vi "Solve_Correspondance_Problem-5.vi"(0 "[IN] Indicies of Po\nints Inside Trks":i32[](array[numeric]), 1 "[IN] Subtracks":T3(array[cluster]), 3 "[IN] Still connected\ntracks in group":T2, 5 "[IN] Indicies of all \nAffected Tracks \n(initial point = 0)":i32[](array[numeric]), 7 "[IN] Index of Optimal \nSubtrack Splitting Case":i32, 9 "[IN] Optimal solution \nfor Merging Case":i32[](array[numeric]), 11 "error IN":errorcluster, 12 "[IN] Status of 1st \nProblem Point":i16) -> (4 "[OUT] Clusters for Re\nconstructed Tracks":T1, 15 "error OUT":errorcluster)   [LabVIEW 2013]
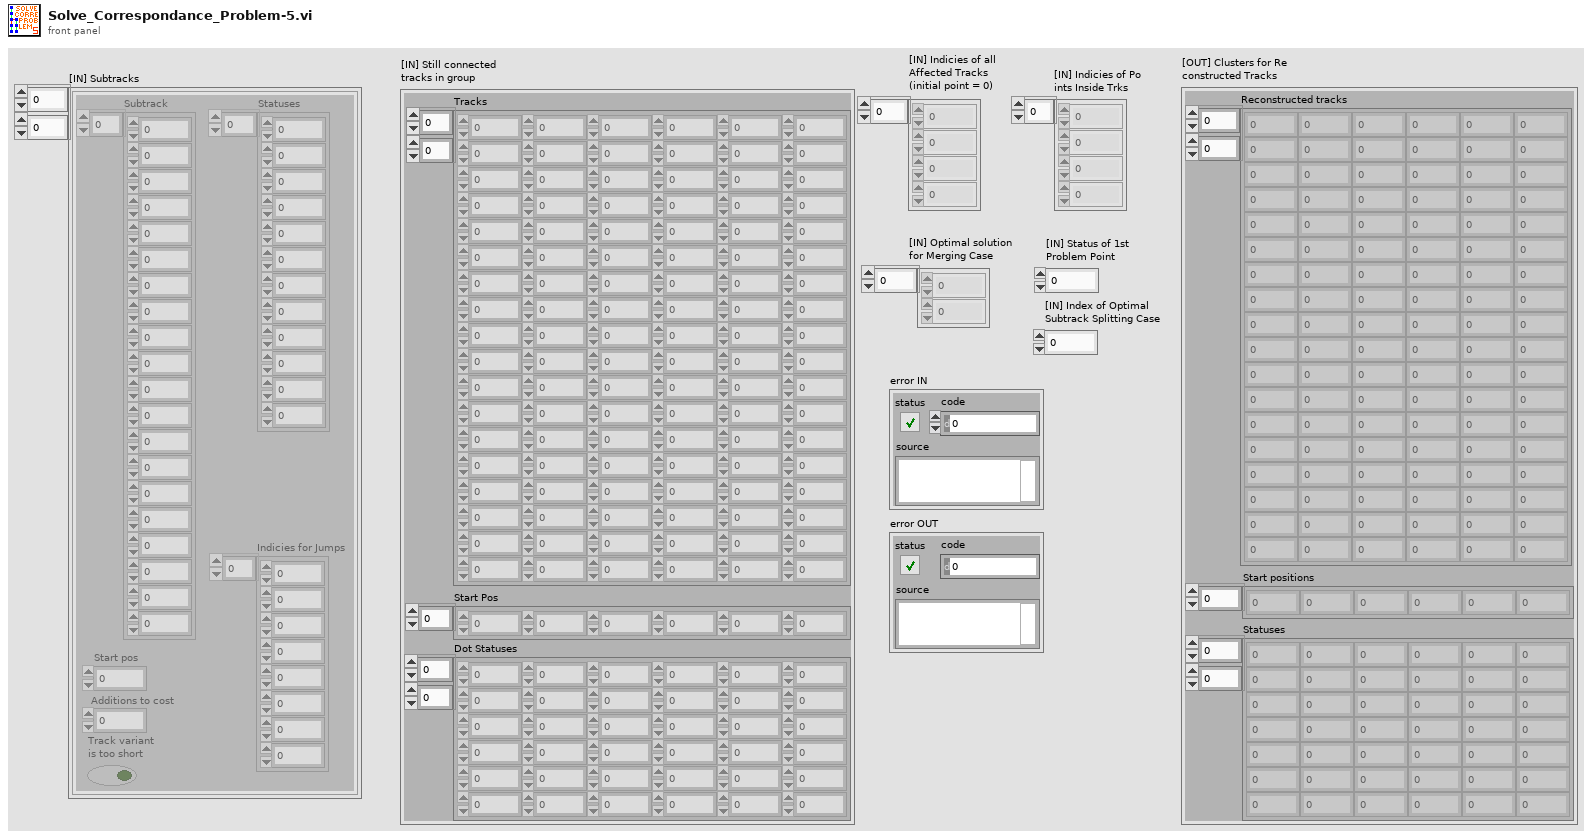
[diagram p1: front panel]
types:
  T1 = cluster{"Reconstructed tracks":dbl[][], "Start positions":i32[], "Statuses":i16[][]}
  T2 = cluster{"Tracks":dbl[][], "Start Pos":i32[], "Dot Statuses":i16[][]}
  T3 = cluster{"Subtrack":dbl[], "Statuses":i16[], "Start pos":i32, "Additions to cost":i8, "Track variant \nis too short":bool, "Indicies for Jumps":i32[]}[][]
  T4 = cluster{"Subtrack":dbl[], "Statuses":i16[], "Start pos":i32, "Additions to cost":i8, "Track variant \nis too short":bool, "Indicies for Jumps":i32[]}[]
  T5 = cluster{"Subtrack":dbl[], "Statuses":i16[], "Start pos":i32, "Additions to cost":i8, "Track variant \nis too short":bool, "Indicies for Jumps":i32[]}
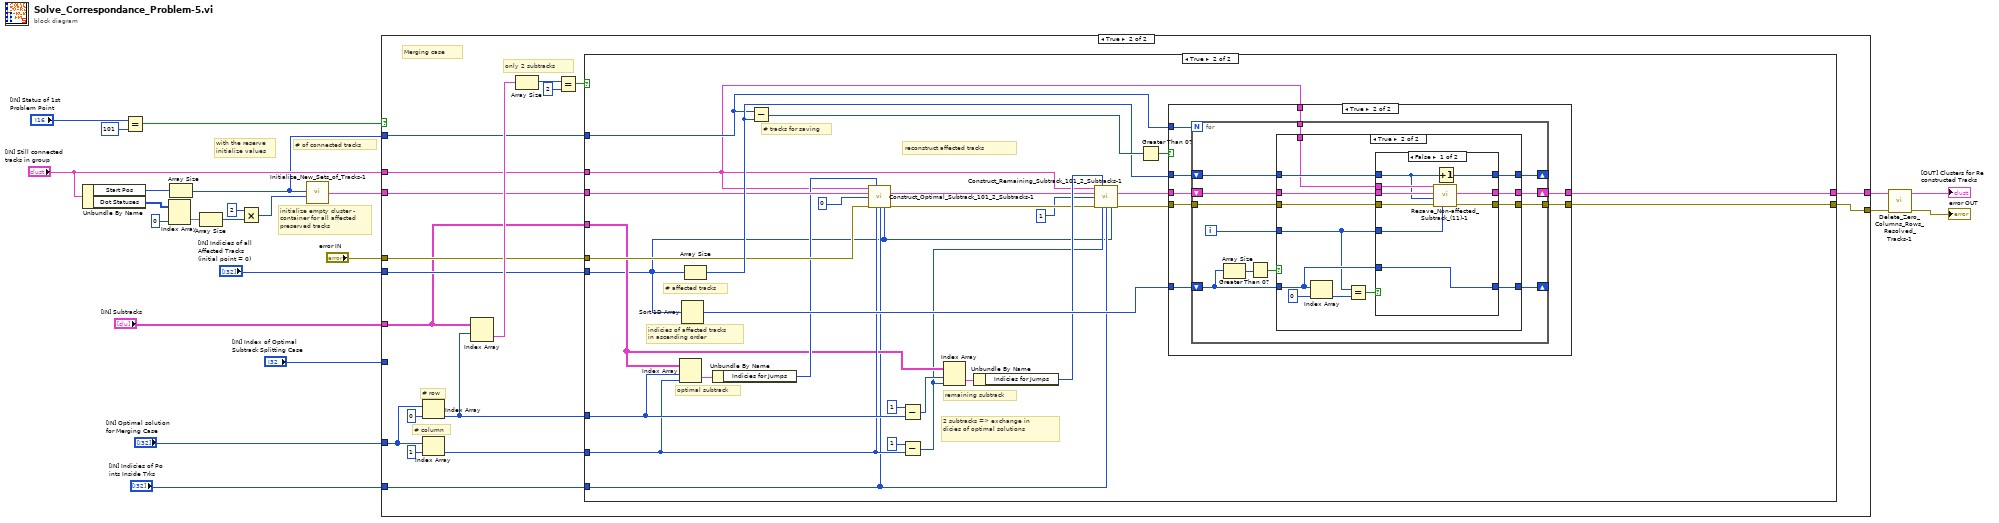
[diagram p0: block diagram]
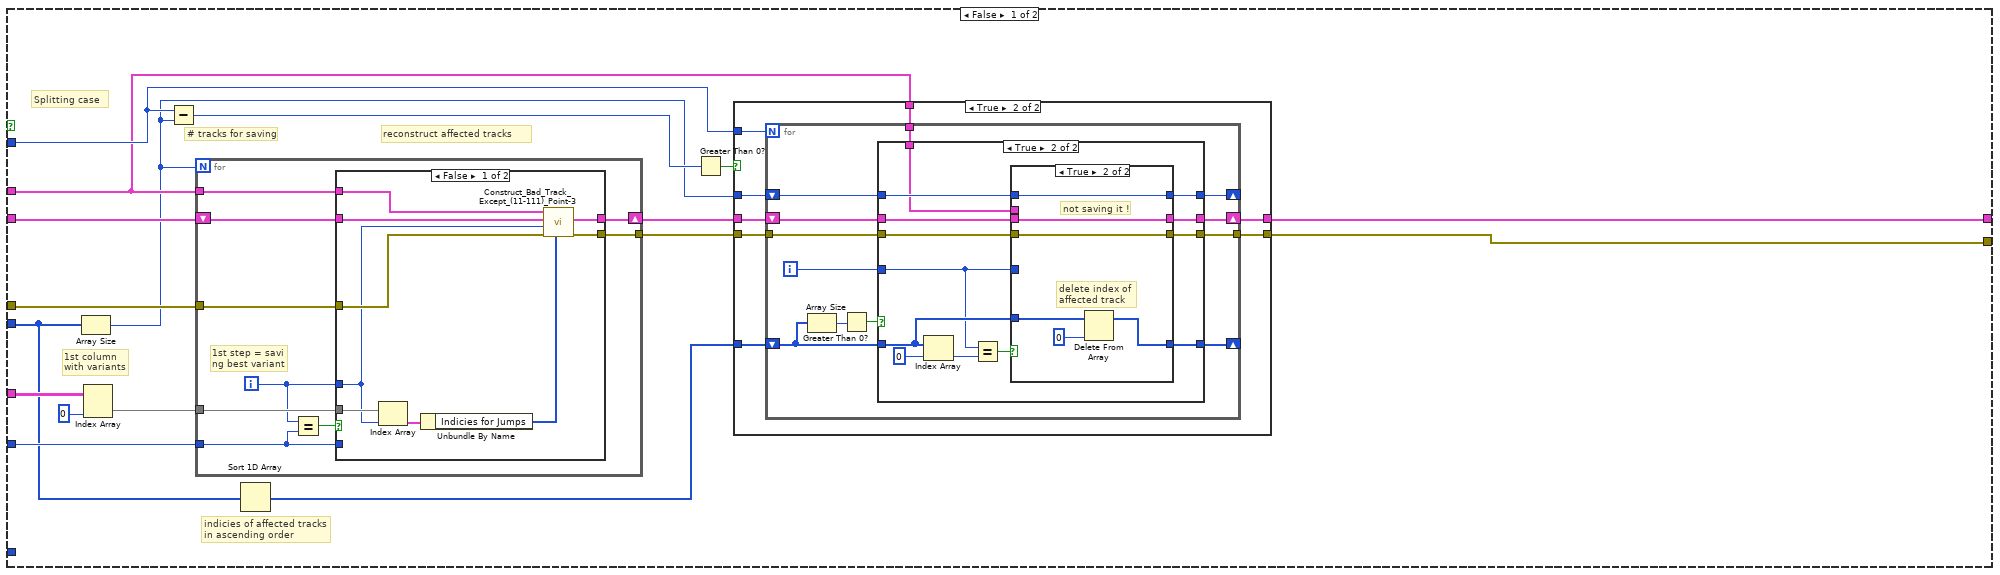
[diagram p2: hidden frame]
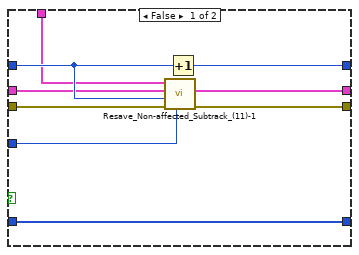
[diagram p4: hidden frame]
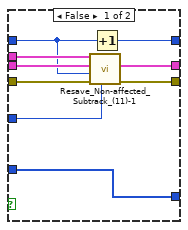
[diagram p5: hidden frame]
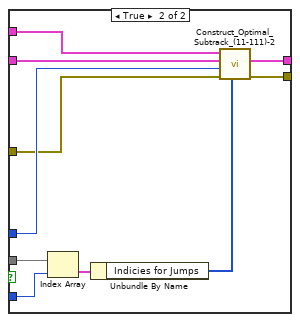
[diagram p6: hidden frame]
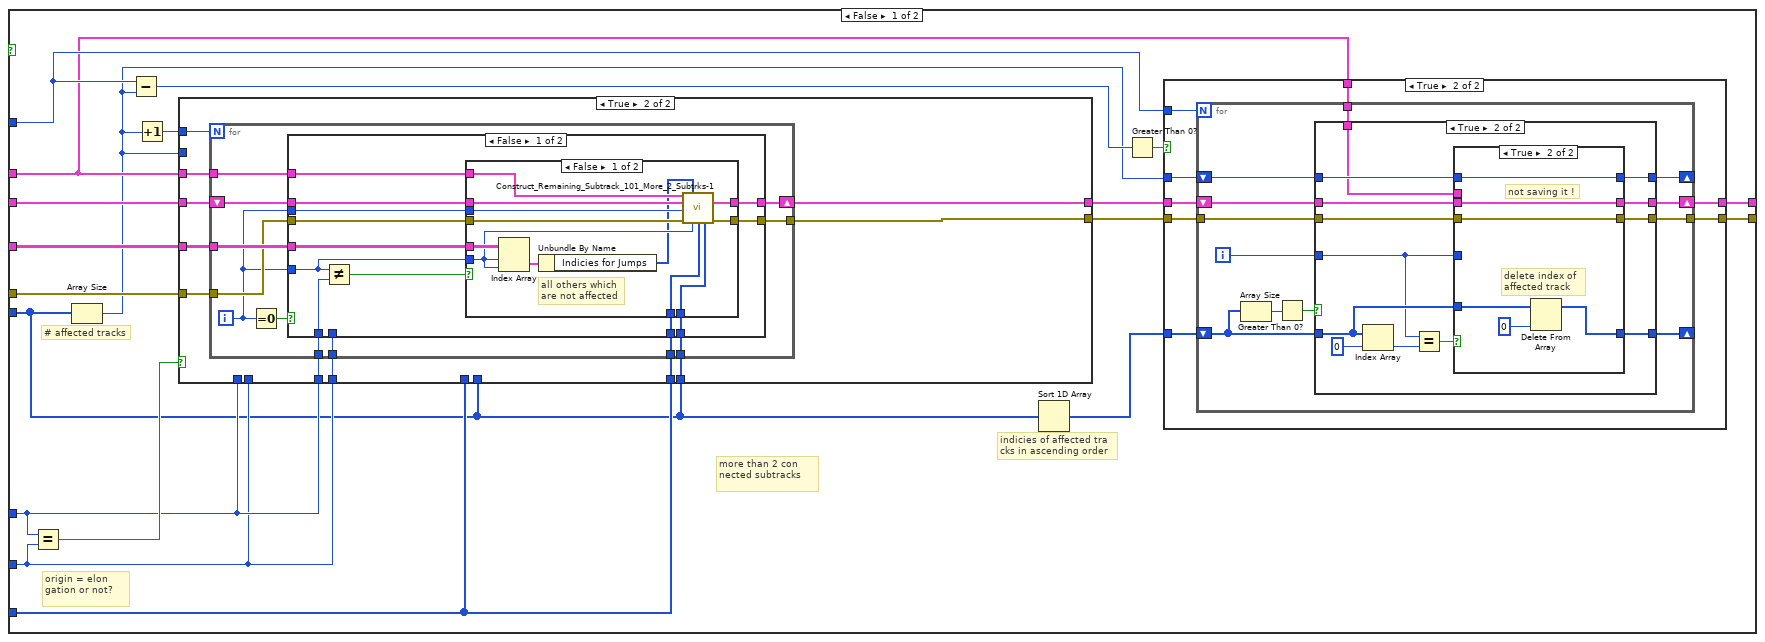
[diagram p7: hidden frame]
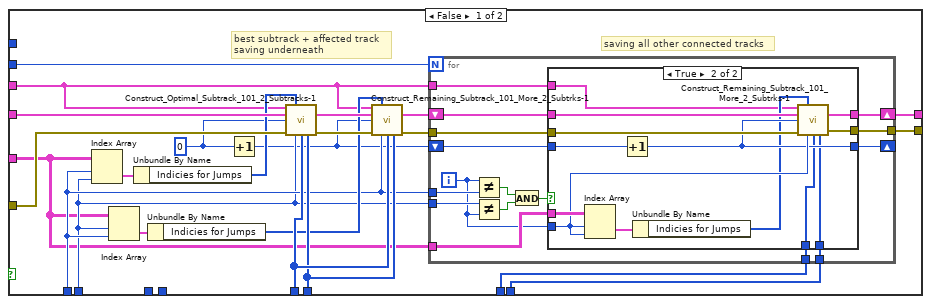
[diagram p8: hidden frame]
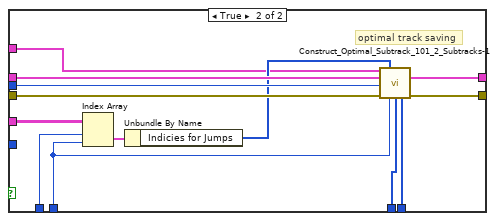
[diagram p11: hidden frame]
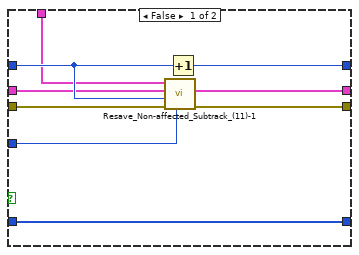
[diagram p13: hidden frame]
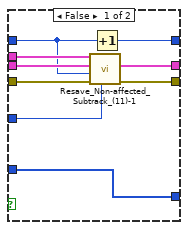
[diagram p14: hidden frame]
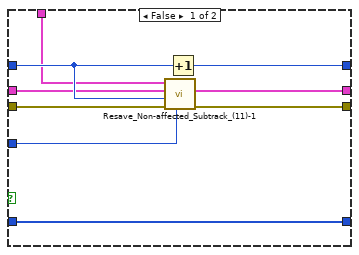
[diagram p16: hidden frame]
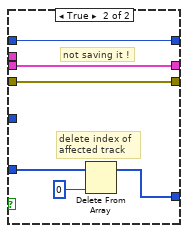
[diagram p17: hidden frame]
diagram:
  # "# of connected tracks"
  # "with the reserve\ninitialize values"
  # "initialize empty cluster - \ncontainer for all affected\npreserved tracks"
  n1 = Unbundle By Name("[IN] Still connected\ntracks in group") -> ("Start Pos"=w19:i32[], "Dot Statuses"=w8:i16[][])
  n2 = Equal?(x="[IN] Status of 1st \nProblem Point", y=i16 101) -> (x = y?=w21:bool)
  n3 = Index Array(array=w8, index (col)=0 ("disabled index (col)")) -> (element=w17:i16[])  [unwired: 1 in]
  n4 = Array Size(array=w19) -> (size(s)=w9:i32)
  n5 = Array Size(array=w17) -> (size(s)=w16:i32)
  n6 = Multiply(x=2, y=w16) -> (x*y=w7:i32)
  n7 = call "Initialize_New_Sets_of_Tracks-1.vi"("[IN] # of Eleme\nnts in New Tracks"=w7, "[IN] # previously \nconnected tracks"=w9) -> ("[OUT] Clusters for Re\nconstructed Tracks"=w14:T1)  [unwired: 4 in]
  n8 = case shown="True" w21 {
    tunnel: "[IN] Still connected\ntracks in group" -> [w27 w135]
    tunnel: w14 -> [w38 w138]
    tunnel: "[IN] Subtracks" -> [w40 w130]
    tunnel: "[IN] Indicies of all \nAffected Tracks \n(initial point = 0)" -> [w29 w136]
    tunnel: "[IN] Index of Optimal \nSubtrack Splitting Case" -> [w36 _]
    tunnel: "error IN" -> [w35 w134]
    tunnel: w9 -> [w30 w137]
    tunnel: [w25 w129] -> w6
    tunnel: [w24 w128] -> w5
    tunnel: "[IN] Optimal solution \nfor Merging Case" -> [_ w143]
    tunnel: "[IN] Indicies of Po\nints Inside Trks" -> [_ w133]
    frame False {
      # "indicies of affected tracks\nin ascending order"
      # "# tracks for saving"
      # "reconstruct affected tracks"
      # "1st column \nwith variants"
      # "Splitting case"
      n9 = Array Size(array=w29) -> (size(s)=w26:i32)
      n10 = Index Array(array=w40, index (col)=0 ("disabled index (col)")) -> (element=w37:T4)  [unwired: 1 in]
      n11 = Subtract(x=w30, y=w26) -> (x-y=w31:i32)
      n12 = for {
        N: w26 -> [_]
        shift-right: [w103] -> w34
        shift-left: w38 -> [w108]
        tunnel: w27 -> [w107]
        tunnel: w37 -> [w105]
        tunnel: w36 -> [w101]
        tunnel: w35 -> [w106]
        tunnel: [w104] -> w33
        i -> [w102]
        # "1st step = savi\nng best variant"
        n13 = Equal?(x=w102, y=w101) -> (x = y?=w100:bool)
        n14 = case shown="False" w100 {
          tunnel: w108 -> [w117 w123]
          tunnel: w107 -> [w116 w124]
          tunnel: w106 -> [w113 w121]
          tunnel: w102 -> [w109 w122]
          tunnel: w105 -> [w115 w127]
          tunnel: w101 -> [_ w126]
          tunnel: [w111 w118] -> w103
          tunnel: [w110 w119] -> w104
          frame False {
            n15 = Index Array(array=w115, index=w109) -> (element=w114:T5)
            n16 = Unbundle By Name(w114) -> ("Indicies for Jumps"=w112:i32[])
            n17 = call "Construct_Bad_Track_Except_(11-111)_Point-3.vi"("[IN] Indexes for Jumps"=w112, "error IN"=w113, "[IN] Index of recon\nstructed tracks"=w109, "[IN] Clusters for Re\nconstructed Tracks"=w117, "[IN] Still connected\ntracks in group"=w116) -> ("error OUT"=w110:errorcluster, "[OUT] Clusters for Re\nconstructed Tracks"=w111:T1)  [unwired: 5 in]
          }
          frame True {
            n18 = Index Array(array=w127, index=w126) -> (element=w125:T5)
            n19 = Unbundle By Name(w125) -> ("Indicies for Jumps"=w120:i32[])
            n20 = call "Construct_Optimal_Subtrack_(11-111)-2.vi"("[IN] Indexes for Jumps"=w120, "error IN"=w121, "[IN] Index of recon\nstructed tracks"=w122, "[IN] Clusters for Re\nconstructed Tracks"=w123, "[IN] Still connected\ntracks in group"=w124) -> ("error OUT"=w119:errorcluster, "[OUT] Clusters for Re\nconstructed Tracks"=w118:T1)  [unwired: 5 in]
          }
        }
      }
      n21 = Sort 1D Array(array=w29) -> (sorted array=w28:i32[])
      n22 = Greater Than 0?(x=w31) -> (x > 0?=w32:bool)
      n23 = case shown="True" w32 {
        tunnel: w34 -> [w42 w48]
        tunnel: w33 -> [w41 w47]
        tunnel: w30 -> [_ w50]
        tunnel: w28 -> [_ w49]
        tunnel: w27 -> [_ w45]
        tunnel: w26 -> [_ w46]
        tunnel: [w41 w44] -> w24
        tunnel: [w42 w43] -> w25
        frame False {
        }
        frame True {
          n24 = for {
            N: w50 -> [_]
            shift-right: [w51] -> _
            shift-left: w49 -> [w52]
            shift-right: [w54] -> w43
            shift-left: w48 -> [w58]
            tunnel: w47 -> [w57]
            shift-right: [w56] -> _
            shift-left: w46 -> [w59]
            tunnel: w45 -> [w55]
            tunnel: [w53] -> w44
            i -> [w60]
            n25 = Array Size(array=w52) -> (size(s)=w62:i32)
            n26 = Greater Than 0?(x=w62) -> (x > 0?=w61:bool)
            n27 = case shown="True" w61 {
              tunnel: w60 -> [w71 w72]
              tunnel: w59 -> [w70 w79]
              tunnel: w58 -> [w69 w81]
              tunnel: w57 -> [w67 w80]
              tunnel: [w68 w76] -> w56
              tunnel: w55 -> [w66 w73]
              tunnel: [w65 w78] -> w54
              tunnel: [w64 w77] -> w53
              tunnel: w52 -> [w63 w75]
              tunnel: [w63 w74] -> w51
              frame False {
                n28 = call "Resave_Non-affected_Subtrack_(11)-1.vi"("[IN] Index for Not\nAffected Track"=w71, "error IN"=w67, "[IN] Index of recon\nstructed tracks"=w70, "[IN] Clusters for Re\nconstructed Tracks"=w69, "[IN] Still connected\ntracks in group"=w66) -> ("error OUT"=w64:errorcluster, "[OUT] Clusters for Re\nconstructed Tracks"=w65:T1)  [unwired: 5 in]
                n29 = Increment(x=w70) -> (x+1=w68:i32)
              }
              frame True {
                n30 = Index Array(array=w75, index=0) -> (element=w83:i32)
                n31 = Equal?(x=w72, y=w83) -> (x = y?=w82:bool)
                n32 = case shown="True" w82 {
                  tunnel: w81 -> [w92 w99]
                  tunnel: w80 -> [w90 w98]
                  tunnel: w79 -> [w86 w97]
                  tunnel: [w88 w99] -> w78
                  tunnel: [w87 w98] -> w77
                  tunnel: [w89 w97] -> w76
                  tunnel: w75 -> [w93 w96]
                  tunnel: [w93 w94] -> w74
                  tunnel: w73 -> [w91 _]
                  tunnel: w72 -> [w85 _]
                  frame False {
                    n33 = call "Resave_Non-affected_Subtrack_(11)-1.vi"("[IN] Index for Not\nAffected Track"=w85, "error IN"=w90, "[IN] Index of recon\nstructed tracks"=w86, "[IN] Clusters for Re\nconstructed Tracks"=w92, "[IN] Still connected\ntracks in group"=w91) -> ("error OUT"=w87:errorcluster, "[OUT] Clusters for Re\nconstructed Tracks"=w88:T1)  [unwired: 5 in]
                    n34 = Increment(x=w86) -> (x+1=w89:i32)
                  }
                  frame True {
                    # "not saving it !"
                    # "delete index of \naffected track"
                    n35 = Delete From Array(array=w96, index=0) -> (array with subset deleted=w94:i32[])  [unwired: 1 in, 1 out]
                  }
                }
              }
            }
          }
        }
      }
    }
    frame True {
      # "Merging case"
      # "only 2 subtracks"
      # "# column"
      # "# row"
      n36 = Index Array(array=w143, index=0) -> (element=w131:i32)
      n37 = Index Array(array=w143, index=1) -> (element=w132:i32)
      n38 = Index Array(array=w130, index (row)=w131) -> (element=w142:T4)  [unwired: 1 in]
      n39 = Array Size(array=w142) -> (size(s)=w141:i32)
      n40 = Equal?(x=w141, y=2) -> (x = y?=w139:bool)
      n41 = case shown="True" w139 {
        tunnel: w138 -> [w156 w364]
        tunnel: w135 -> [w157 w348]
        tunnel: w137 -> [w161 w365]
        tunnel: w136 -> [w147 w343]
        tunnel: w134 -> [w158 w362]
        tunnel: w133 -> [w149 w344]
        tunnel: w132 -> [w150 w354]
        tunnel: w131 -> [w151 w356]
        tunnel: w130 -> [w155 w353]
        tunnel: [w163 w361] -> w129
        tunnel: [w162 w360] -> w128
        frame False {
          # "indicies of affected tra\ncks in ascending order"
          # "origin = elon\ngation or not?"
          # "# affected tracks"
          # "more than 2 con\nnected subtracks"
          n42 = Equal?(x=w151, y=w150) -> (x = y?=w159:bool)
          n43 = Array Size(array=w147) -> (size(s)=w148:i32)
          n44 = Subtract(x=w161, y=w148) -> (x-y=w160:i32)
          n45 = Increment(x=w148) -> (x+1=w154:i32)
          n46 = case shown="True" w159 {
            tunnel: w158 -> [w185 w230]
            tunnel: w154 -> [_ w229]
            tunnel: w157 -> [w170 w228]
            tunnel: w156 -> [w186 w227]
            tunnel: w155 -> [w171 w226]
            tunnel: w151 -> [_ w225]
            tunnel: w150 -> [_ w224]
            tunnel: w147 -> [w165 w223]
            tunnel: w149 -> [w166 w222]
            tunnel: [w168 w221] -> w153
            tunnel: [w169 w220] -> w152
            tunnel: w151 -> [w173 _]
            tunnel: w150 -> [w172 _]
            tunnel: w149 -> [w180 _]
            tunnel: w147 -> [w179 _]
            tunnel: w148 -> [w176 _]
            frame False {
              w181 = 0 ("[IN] Index of recon\nstructed tracks")
              # "saving all other connected tracks"
              # "best subtrack + affected track \nsaving underneath"
              n47 = Index Array(array=w171, index (row)=w173, index (col)=w172) -> (element=w187:T5)
              n48 = Index Array(array=w171, index (row)=w172, index (col)=w173) -> (element=w178:T5)
              n49 = Unbundle By Name(w187) -> ("Indicies for Jumps"=w184:i32[])
              n50 = Unbundle By Name(w178) -> ("Indicies for Jumps"=w177:i32[])
              n51 = Increment(x=w181) -> (x+1=w167:i32)
              n52 = call "Construct_Optimal_Subtrack_101_2_Subtracks-1.vi"("[IN] Still connected\ntracks in group"=w170, "[IN] Indexes for Jumps"=w184, "[IN] Clusters for Re\nconstructed Tracks"=w186, "[IN] Index of recon\nstructed tracks"=w181, "error IN"=w185, "[IN] # column of op\ntimal elongation"=w172, "[IN] Indicies of Po\nints Inside Trks"=w180, "[IN] Indicies of all \nAffected Tracks \n(initial point = 0)"=w179) -> ("[OUT] Clusters for Re\nconstructed Tracks"=w183:T1, "error OUT"=w182:errorcluster)  [unwired: 6 in]
              n53 = call "Construct_Remaining_Subtrack_101_More_2_Subtrks-1.vi"("[IN] Still connected\ntracks in group"=w170, "[IN] Indexes for Jumps"=w177, "[IN] Clusters for Re\nconstructed Tracks"=w183, "[IN] Index of recon\nstructed tracks"=w167, "error IN"=w182, "[IN] # column of re\nmaining elongation"=w173, "[IN] Indicies of Po\nints Inside Trks"=w180, "[IN] Indicies of all \nAffected Tracks \n(initial point = 0)"=w179) -> ("[OUT] Clusters for Re\nconstructed Tracks"=w175:T1, "error OUT"=w174:errorcluster)  [unwired: 6 in]
              n54 = for {
                N: w176 -> [_]
                shift-right: [w194] -> w169
                shift-left: w175 -> [w196]
                tunnel: w174 -> [w195]
                tunnel: w173 -> [w203]
                tunnel: w172 -> [w202]
                tunnel: w171 -> [w198]
                tunnel: w170 -> [w197]
                tunnel: [w193] -> w168
                shift-right: [w190] -> _
                shift-left: w167 -> [w191]
                tunnel: w166 -> [w189]
                tunnel: w165 -> [w188]
                i -> [w192]
                n55 = Not Equal?(x=w192, y=w203) -> (x != y?=w201:bool)
                n56 = Not Equal?(x=w202, y=w192) -> (x != y?=w200:bool)
                n57 = And(x=w201, y=w200) -> (x .and. y?=w199:bool)
                n58 = case shown="True" w199 {
                  tunnel: w198 -> [_ w219]
                  tunnel: w192 -> [_ w215]
                  tunnel: w197 -> [_ w207]
                  tunnel: w196 -> [w206 w217]
                  tunnel: w195 -> [w205 w213]
                  tunnel: [w206 w216] -> w194
                  tunnel: [w205 w214] -> w193
                  tunnel: w191 -> [w204 w212]
                  tunnel: [w204 w211] -> w190
                  tunnel: w189 -> [_ w209]
                  tunnel: w188 -> [_ w208]
                  frame False {
                  }
                  frame True {
                    n59 = Index Array(array=w219, index (row)=w215, index (col)=w215) -> (element=w218:T5)
                    n60 = Increment(x=w212) -> (x+1=w211:i32)
                    n61 = Unbundle By Name(w218) -> ("Indicies for Jumps"=w210:i32[])
                    n62 = call "Construct_Remaining_Subtrack_101_More_2_Subtrks-1.vi"("[IN] Still connected\ntracks in group"=w207, "[IN] Indexes for Jumps"=w210, "[IN] Clusters for Re\nconstructed Tracks"=w217, "[IN] Index of recon\nstructed tracks"=w211, "error IN"=w213, "[IN] # column of re\nmaining elongation"=w215, "[IN] Indicies of Po\nints Inside Trks"=w209, "[IN] Indicies of all \nAffected Tracks \n(initial point = 0)"=w208) -> ("[OUT] Clusters for Re\nconstructed Tracks"=w216:T1, "error OUT"=w214:errorcluster)  [unwired: 6 in]
                  }
                }
              }
            }
            frame True {
              n63 = for {
                N: w229 -> [_]
                tunnel: w230 -> [w237]
                tunnel: w228 -> [w241]
                shift-right: [w233] -> w220
                shift-left: w227 -> [w240]
                tunnel: w226 -> [w239]
                tunnel: w225 -> [w238]
                tunnel: w224 -> [w236]
                tunnel: w223 -> [w235]
                tunnel: w222 -> [w234]
                tunnel: [w232] -> w221
                i -> [w231]
                n64 = Equal To 0?(x=w231) -> (x = 0?=w242:bool)
                n65 = case shown="False" w242 {
                  tunnel: w231 -> [w250 w281]
                  tunnel: w241 -> [w246 w274]
                  tunnel: w240 -> [w251 w280]
                  tunnel: w239 -> [w252 w279]
                  tunnel: w238 -> [w254 w278]
                  tunnel: w237 -> [w249 w277]
                  tunnel: w236 -> [_ w273]
                  tunnel: w235 -> [w244 w272]
                  tunnel: w234 -> [w243 w271]
                  tunnel: [w247 w270] -> w233
                  tunnel: [w248 w269] -> w232
                  tunnel: w231 -> [w245 _]
                  frame False {
                    n66 = Not Equal?(x=w245, y=w254) -> (x != y?=w253:bool)
                    n67 = case shown="False" w253 {
                      tunnel: w252 -> [w261 _]
                      tunnel: w251 -> [w266 w267]
                      tunnel: w250 -> [w256 _]
                      tunnel: w249 -> [w264 w268]
                      tunnel: [w263 w268] -> w248
                      tunnel: [w262 w267] -> w247
                      tunnel: w246 -> [w265 _]
                      tunnel: w245 -> [w257 _]
                      tunnel: w244 -> [w259 _]
                      tunnel: w243 -> [w258 _]
                      frame False {
                        # "all others which\nare not affected"
                        n68 = Index Array(array=w261, index (row)=w257, index (col)=w257) -> (element=w260:T5)
                        n69 = Unbundle By Name(w260) -> ("Indicies for Jumps"=w255:i32[])
                        n70 = call "Construct_Remaining_Subtrack_101_More_2_Subtrks-1.vi"("[IN] Still connected\ntracks in group"=w265, "[IN] Indexes for Jumps"=w255, "[IN] Clusters for Re\nconstructed Tracks"=w266, "[IN] Index of recon\nstructed tracks"=w256, "error IN"=w264, "[IN] # column of re\nmaining elongation"=w257, "[IN] Indicies of Po\nints Inside Trks"=w258, "[IN] Indicies of all \nAffected Tracks \n(initial point = 0)"=w259) -> ("[OUT] Clusters for Re\nconstructed Tracks"=w262:T1, "error OUT"=w263:errorcluster)  [unwired: 6 in]
                      }
                      frame True {
                      }
                    }
                  }
                  frame True {
                    # "optimal track saving"
                    n71 = Index Array(array=w279, index (row)=w278, index (col)=w273) -> (element=w276:T5)
                    n72 = Unbundle By Name(w276) -> ("Indicies for Jumps"=w275:i32[])
                    n73 = call "Construct_Optimal_Subtrack_101_2_Subtracks-1.vi"("[IN] Still connected\ntracks in group"=w274, "[IN] Indexes for Jumps"=w275, "[IN] Clusters for Re\nconstructed Tracks"=w280, "[IN] Index of recon\nstructed tracks"=w281, "error IN"=w277, "[IN] # column of op\ntimal elongation"=w273, "[IN] Indicies of Po\nints Inside Trks"=w271, "[IN] Indicies of all \nAffected Tracks \n(initial point = 0)"=w272) -> ("[OUT] Clusters for Re\nconstructed Tracks"=w270:T1, "error OUT"=w269:errorcluster)  [unwired: 6 in]
                  }
                }
              }
            }
          }
          n74 = Sort 1D Array(array=w147) -> (sorted array=w146:i32[])
          n75 = Greater Than 0?(x=w160) -> (x > 0?=w164:bool)
          n76 = case shown="True" w164 {
            tunnel: w152 -> [w283 w289]
            tunnel: w153 -> [w282 w288]
            tunnel: w161 -> [_ w291]
            tunnel: w146 -> [_ w290]
            tunnel: w157 -> [_ w286]
            tunnel: w148 -> [_ w287]
            tunnel: [w282 w285] -> w162
            tunnel: [w283 w284] -> w163
            frame False {
            }
            frame True {
              n77 = for {
                N: w291 -> [_]
                shift-right: [w292] -> _
                shift-left: w290 -> [w293]
                shift-right: [w295] -> w284
                shift-left: w289 -> [w299]
                tunnel: w288 -> [w298]
                shift-right: [w297] -> _
                shift-left: w287 -> [w300]
                tunnel: w286 -> [w296]
                tunnel: [w294] -> w285
                i -> [w301]
                n78 = Array Size(array=w293) -> (size(s)=w303:i32)
                n79 = Greater Than 0?(x=w303) -> (x > 0?=w302:bool)
                n80 = case shown="True" w302 {
                  tunnel: w301 -> [w312 w313]
                  tunnel: w300 -> [w311 w320]
                  tunnel: w299 -> [w310 w322]
                  tunnel: w298 -> [w308 w321]
                  tunnel: [w309 w317] -> w297
                  tunnel: w296 -> [w307 w314]
                  tunnel: [w306 w319] -> w295
                  tunnel: [w305 w318] -> w294
                  tunnel: w293 -> [w304 w316]
                  tunnel: [w304 w315] -> w292
                  frame False {
                    n81 = call "Resave_Non-affected_Subtrack_(11)-1.vi"("[IN] Index for Not\nAffected Track"=w312, "error IN"=w308, "[IN] Index of recon\nstructed tracks"=w311, "[IN] Clusters for Re\nconstructed Tracks"=w310, "[IN] Still connected\ntracks in group"=w307) -> ("error OUT"=w305:errorcluster, "[OUT] Clusters for Re\nconstructed Tracks"=w306:T1)  [unwired: 5 in]
                    n82 = Increment(x=w311) -> (x+1=w309:i32)
                  }
                  frame True {
                    n83 = Index Array(array=w316, index=0) -> (element=w324:i32)
                    n84 = Equal?(x=w313, y=w324) -> (x = y?=w323:bool)
                    n85 = case shown="True" w323 {
                      tunnel: w322 -> [w333 w340]
                      tunnel: w321 -> [w331 w339]
                      tunnel: w320 -> [w327 w338]
                      tunnel: [w329 w340] -> w319
                      tunnel: [w328 w339] -> w318
                      tunnel: [w330 w338] -> w317
                      tunnel: w316 -> [w334 w337]
                      tunnel: [w334 w335] -> w315
                      tunnel: w314 -> [w332 _]
                      tunnel: w313 -> [w326 _]
                      frame False {
                        n86 = call "Resave_Non-affected_Subtrack_(11)-1.vi"("[IN] Index for Not\nAffected Track"=w326, "error IN"=w331, "[IN] Index of recon\nstructed tracks"=w327, "[IN] Clusters for Re\nconstructed Tracks"=w333, "[IN] Still connected\ntracks in group"=w332) -> ("error OUT"=w328:errorcluster, "[OUT] Clusters for Re\nconstructed Tracks"=w329:T1)  [unwired: 5 in]
                        n87 = Increment(x=w327) -> (x+1=w330:i32)
                      }
                      frame True {
                        # "not saving it !"
                        # "delete index of \naffected track"
                        n88 = Delete From Array(array=w337, index=0) -> (array with subset deleted=w335:i32[])  [unwired: 1 in, 1 out]
                      }
                    }
                  }
                }
              }
            }
          }
        }
        frame True {
          # "remaining subtrack"
          # "optimal subtrack"
          # "2 subtracks => exchange in\ndicies of optimal solutions"
          # "indicies of affected tracks\nin ascending order"
          # "# tracks for saving"
          # "reconstruct affected tracks"
          # "# affected tracks"
          n89 = Index Array(array=w353, index (row)=w356, index (col)=w354) -> (element=w359:T5)
          n90 = Sort 1D Array(array=w343) -> (sorted array=w367:i32[])
          n91 = Array Size(array=w343) -> (size(s)=w366:i32)
          n92 = Unbundle By Name(w359) -> ("Indicies for Jumps"=w358:i32[])
          n93 = Subtract(x=w365, y=w366) -> (x-y=w368:i32)
          n94 = call "Construct_Optimal_Subtrack_101_2_Subtracks-1.vi"("[IN] Still connected\ntracks in group"=w348, "[IN] Indexes for Jumps"=w358, "[IN] Clusters for Re\nconstructed Tracks"=w364, "[IN] Index of recon\nstructed tracks"=0 ("[IN] Index of recon\nstructed tracks"), "error IN"=w362, "[IN] # column of op\ntimal elongation"=w354, "[IN] Indicies of Po\nints Inside Trks"=w344, "[IN] Indicies of all \nAffected Tracks \n(initial point = 0)"=w343) -> ("[OUT] Clusters for Re\nconstructed Tracks"=w350:T1, "error OUT"=w349:errorcluster)  [unwired: 6 in]
          n95 = Subtract(x=1, y=w356) -> (x-y=w346:i32)
          n96 = Subtract(x=1, y=w354) -> (x-y=w345:i32)
          n97 = Index Array(array=w353, index (row)=w346, index (col)=w345) -> (element=w352:T5)
          n98 = Unbundle By Name(w352) -> ("Indicies for Jumps"=w351:i32[])
          n99 = call "Construct_Remaining_Subtrack_101_2_Subtracks-1.vi"("[IN] Still connected\ntracks in group"=w348, "[IN] Indexes for Jumps"=w351, "[IN] Clusters for Re\nconstructed Tracks"=w350, "[IN] Index of recon\nstructed tracks"=1 ("[IN] Index of recon\nstructed tracks"), "error IN"=w349, "[IN] # column of re\nmaining elongation"=w345, "[IN] Indicies of Po\nints Inside Trks"=w344, "[IN] Indicies of all \nAffected Tracks \n(initial point = 0)"=w343) -> ("[OUT] Clusters for Re\nconstructed Tracks"=w342:T1, "error OUT"=w341:errorcluster)  [unwired: 6 in]
          n100 = Greater Than 0?(x=w368) -> (x > 0?=w369:bool)
          n101 = case shown="True" w369 {
            tunnel: w342 -> [w371 w377]
            tunnel: w341 -> [w370 w376]
            tunnel: w365 -> [_ w379]
            tunnel: w367 -> [_ w378]
            tunnel: w348 -> [_ w374]
            tunnel: w366 -> [_ w375]
            tunnel: [w370 w373] -> w360
            tunnel: [w371 w372] -> w361
            frame False {
            }
            frame True {
              n102 = for {
                N: w379 -> [_]
                shift-right: [w380] -> _
                shift-left: w378 -> [w381]
                shift-right: [w383] -> w372
                shift-left: w377 -> [w387]
                tunnel: w376 -> [w386]
                shift-right: [w385] -> _
                shift-left: w375 -> [w388]
                tunnel: w374 -> [w384]
                tunnel: [w382] -> w373
                i -> [w389]
                n103 = Array Size(array=w381) -> (size(s)=w391:i32)
                n104 = Greater Than 0?(x=w391) -> (x > 0?=w390:bool)
                n105 = case shown="True" w390 {
                  tunnel: w389 -> [w400 w401]
                  tunnel: w388 -> [w399 w408]
                  tunnel: w387 -> [w398 w410]
                  tunnel: w386 -> [w396 w409]
                  tunnel: [w397 w405] -> w385
                  tunnel: w384 -> [w395 w402]
                  tunnel: [w394 w407] -> w383
                  tunnel: [w393 w406] -> w382
                  tunnel: w381 -> [w392 w404]
                  tunnel: [w392 w403] -> w380
                  frame False {
                    n106 = call "Resave_Non-affected_Subtrack_(11)-1.vi"("[IN] Index for Not\nAffected Track"=w400, "error IN"=w396, "[IN] Index of recon\nstructed tracks"=w399, "[IN] Clusters for Re\nconstructed Tracks"=w398, "[IN] Still connected\ntracks in group"=w395) -> ("error OUT"=w393:errorcluster, "[OUT] Clusters for Re\nconstructed Tracks"=w394:T1)  [unwired: 5 in]
                    n107 = Increment(x=w399) -> (x+1=w397:i32)
                  }
                  frame True {
                    n108 = Index Array(array=w404, index=0) -> (element=w412:i32)
                    n109 = Equal?(x=w401, y=w412) -> (x = y?=w411:bool)
                    n110 = case shown="False" w411 {
                      tunnel: w410 -> [w421 w428]
                      tunnel: w409 -> [w419 w427]
                      tunnel: w408 -> [w415 w426]
                      tunnel: [w417 w428] -> w407
                      tunnel: [w416 w427] -> w406
                      tunnel: [w418 w426] -> w405
                      tunnel: w404 -> [w422 w425]
                      tunnel: [w422 w423] -> w403
                      tunnel: w402 -> [w420 _]
                      tunnel: w401 -> [w414 _]
                      frame False {
                        n111 = call "Resave_Non-affected_Subtrack_(11)-1.vi"("[IN] Index for Not\nAffected Track"=w414, "error IN"=w419, "[IN] Index of recon\nstructed tracks"=w415, "[IN] Clusters for Re\nconstructed Tracks"=w421, "[IN] Still connected\ntracks in group"=w420) -> ("error OUT"=w416:errorcluster, "[OUT] Clusters for Re\nconstructed Tracks"=w417:T1)  [unwired: 5 in]
                        n112 = Increment(x=w415) -> (x+1=w418:i32)
                      }
                      frame True {
                        # "not saving it !"
                        # "delete index of \naffected track"
                        n113 = Delete From Array(array=w425, index=0) -> (array with subset deleted=w423:i32[])  [unwired: 1 in, 1 out]
                      }
                    }
                  }
                }
              }
            }
          }
        }
      }
    }
  }
  n114 = call "Delete_Zero_Columns_Rows_Resolved_Tracks-1.vi"("error IN"=w5, "[IN] Clusters for Re\nconstructed Tracks"=w6) -> ("error OUT"=→"error OUT":errorcluster, "[OUT] Clusters for Re\nconstructed Tracks"=→"[OUT] Clusters for Re\nconstructed Tracks":T1)  [unwired: 4 in]
